vi "Initialize Tree Symbols.vi"(8 "error in (no error)":errorcluster, 11 "TreeControl in":refnum<vi>) -> (0 "error out":errorcluster, 3 "TreeControl out":refnum<vi>)   [LabVIEW 2015, in "Shared Variable Custom Device.lvlib"]
uses:
  Shared Variable Custom Device.lvlib
  Shared/Shared Variable Globals.vi
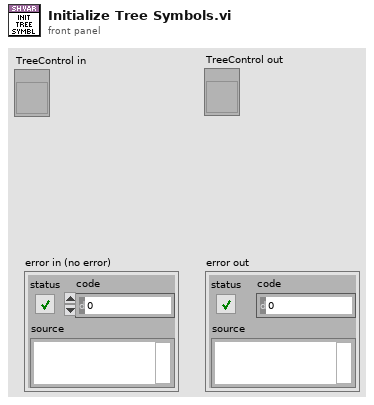
[diagram p1: front panel]
types:
  T1 = typedef "imagedata.ctl" = cluster{"image type":i32, "image depth":i32, "image":u8[], "mask":u8[], "colors":u32[], "Rectangle":cluster{"left":i16, "top":i16, "right":i16, "bottom":i16}}
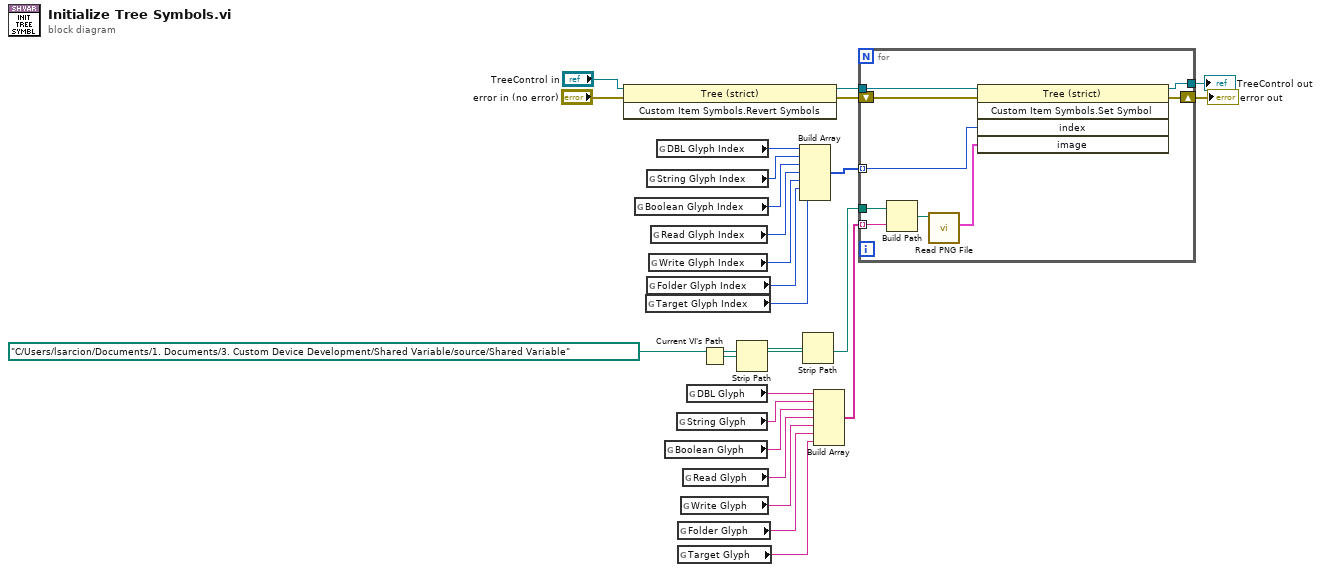
[diagram p0: block diagram]
diagram:
  n1 = invoke class="Tree (strict)" method="Custom Item Symbols.Revert Symbols"(reference="TreeControl in", error in="error in (no error)") -> (reference out=w5:refnum<vi>, error out=w4:errorcluster)  [unwired: 1 in, 1 out]
  n2 = global read "Shared Variable Globals.vi" "Boolean Glyph Index"() -> (w21:i32)
  n3 = global read "Shared Variable Globals.vi" "Target Glyph Index"() -> (w1:i32)
  n4 = global read "Shared Variable Globals.vi" "String Glyph Index"() -> (w20:i32)
  n5 = global read "Shared Variable Globals.vi" "Folder Glyph Index"() -> (w8:i32)
  n6 = global read "Shared Variable Globals.vi" "Write Glyph Index"() -> (w23:i32)
  n7 = global read "Shared Variable Globals.vi" "Read Glyph Index"() -> (w22:i32)
  n8 = global read "Shared Variable Globals.vi" "DBL Glyph Index"() -> (w19:i32)
  n9 = global read "Shared Variable Globals.vi" "Boolean Glyph"() -> (w16:string)
  n10 = global read "Shared Variable Globals.vi" "String Glyph"() -> (w15:string)
  n11 = global read "Shared Variable Globals.vi" "Folder Glyph"() -> (w9:string)
  n12 = global read "Shared Variable Globals.vi" "Target Glyph"() -> (w2:string)
  n13 = global read "Shared Variable Globals.vi" "Write Glyph"() -> (w18:string)
  n14 = global read "Shared Variable Globals.vi" "Read Glyph"() -> (w17:string)
  n15 = global read "Shared Variable Globals.vi" "DBL Glyph"() -> (w14:string)
  n16 = Current VI's Path() -> (path=w13:path)
  n17 = Strip Path(path=w13) -> (stripped path=w12:path)  [unwired: 1 out]
  n18 = Build Array(w19, w20, w21, w22, w23, w8, w1) -> (w25:i32[])
  n19 = Strip Path(path=w12) -> ()  [unwired: 2 out]
  n20 = Build Array(w14, w15, w16, w17, w18, w9, w2) -> (w24:string[])
  n21 = for {
    tunnel: w24 -> [w29] mode=indexing
    tunnel: w25 -> [w31] mode=indexing
    shift-right: [w33] -> w11
    shift-left: w4 -> [w34]
    tunnel: w5 -> [w32]
    tunnel: path "C:/Users/lsarcion/Documents/1. Documents/3. Custom Device Development/Shared Variable/source/Shared Variable" -> [w30]
    tunnel: [w26] -> w10
    n22 = Build Path(base path=w30, name or relative path=w29) -> (appended path=w28:path)
    n23 = call <vilib>:"Read PNG File.vi"("path to PNG file"=w28) -> ("image data"=w27:T1)  [unwired: 8 in, 2 out]
    n24 = invoke on="Invoke Node" class="Tree (strict)" method="Custom Item Symbols.Set Symbol"(reference=w32, error in=w34, "index"=w31, "image"=w27) -> (reference out=w26:refnum<vi>, error out=w33:errorcluster)  [unwired: 1 in, 3 out]
  }
  "error out" <- w11
  "TreeControl out" <- w10
